vi "state_detect.vi"() -> ()   [LabVIEW 2012]
uses:
  <vilib>/DAQmx/create/channels.llb/DAQmx Create Channel (CO-Pulse Generation-Frequency).vi
  <vilib>/DAQmx/configure/timing.llb/DAQmx Timing (Implicit).vi
  <vilib>/Utility/file.llb/Write To Spreadsheet File (DBL).vi
  <vilib>/Analysis/NI_AALBase.lvlib
panel:
  in  "Save data to":path
  out "Fluorescence Before":T1(graph)
  out "Run Number":i32
  out "Total fluorescence with pumping":u32
  out "Total fluorescence without pumping":u32
  out "Optical pumping":bool
  out "Not_opt_pump_dark_runs":i32
  out "opt_pump_dark_runs":i32
  in  "Fluoresence Threshold":u32
  out "No_opt_pump_dark_run_ratio":dbl
  out "Opt_pump_Dark_run_ratio":dbl
  out "Fluorescence After":T2(graph)
  in  "Runs":i32
  in  "stop":bool
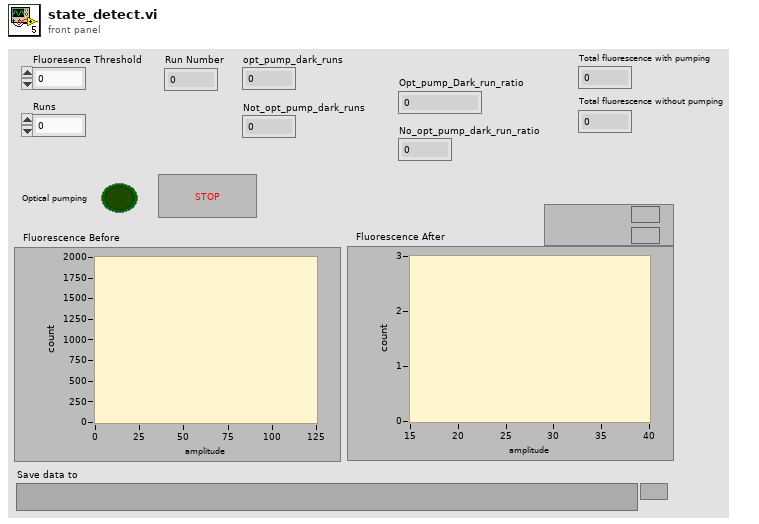
[diagram p1: front panel]
types:
  T1 = cluster{"X Values":dbl[], "Histogram: h(x)":i32[]}
  T2 = cluster{"X Values":dbl[], "Histogram: h(x)":i32[]}[]
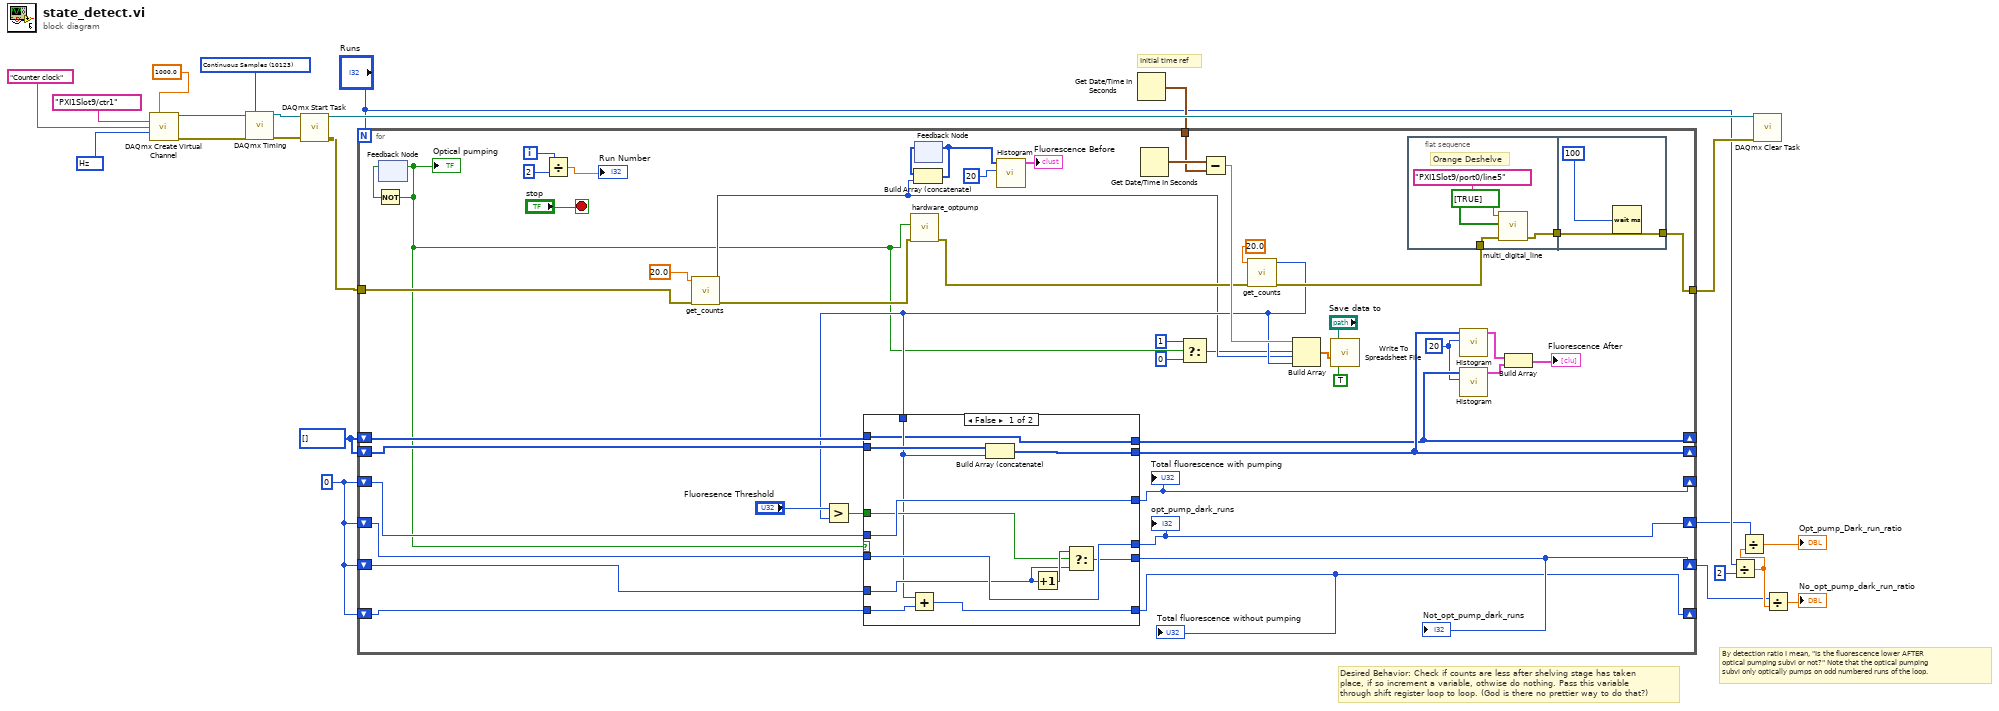
[diagram p0: block diagram]
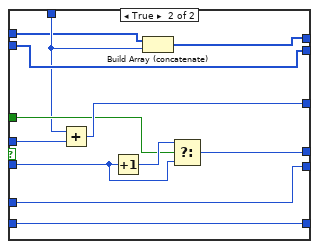
[diagram p2: hidden frame]
diagram:
  w2 = i32[] [] ("initialized array")
  w1 = 0
  w17 = 10123 items=["Finite Samples"=10178, "Continuous Samples"=10123, "Hardware Timed Single Point"=12522] ("sample mode")
  w22 = 10373 items=["Hz"=10373] ("units")
  # "Desired Behavior: Check if counts are less after shelving stage has taken\nplace, if so increment a variable, othwise do nothing. Pass this variable\nthrough shift register loop to loop. (God is there no prettier way to do that?)"
  # "Initial time ref"
  # "By detection ratio I mean, \"Is the fluorescence lower AFTER\noptical pumping subvi or not?\" Note that the optical pumping\nsubvi only optically pumps on odd numbered runs of the loop."
  n1 = call-poly <vilib>:"DAQmx Create Virtual Channel.vi"("frequency"=1000.0 ("rate"), "counter"=tag "PXI1Slot9/ctr1", "name to assign"="Counter clock", "units"=w22) -> ("task out"=w21:refnum<k21>, "error out"=w20:errorcluster)  [unwired: 10 in]
  n2 = call-poly <vilib>:"DAQmx Timing.vi"("task/channels in"=w21, "sample mode"=w17, "error in"=w20) -> ("task out"=w19:refnum<k21>, "error out"=w18:errorcluster)  [unwired: 11 in]
  n3 = call <vilib>:"DAQmx Start Task.vi"("task/channels in"=w19, "error in"=w18) -> ("task out"=w12:refnum<k21>, "error out"=w13:errorcluster)  [unwired: 12 in]
  n4 = Get Date/Time In Seconds() -> (seconds since 1Jan1904=w11:timestamp)
  n5 = for {
    N: "Runs" -> [_]
    tunnel: w13 -> [w63]
    tunnel: w11 -> [w66]
    tunnel: [w59] -> w10
    shift-right: [w42] -> _
    shift-left: w2 -> [w43]
    shift-right: [w40] -> _
    shift-left: w2 -> [w41]
    shift-right: [w55] -> w5
    shift-left: w1 -> [w62]
    shift-right: [w54] -> w7
    shift-left: w1 -> [w61]
    shift-right: [w50] -> _
    shift-left: w1 -> [w52]
    shift-right: [w51] -> _
    shift-left: w1 -> [w53]
    i -> [w48]
    stop <- "stop" stop-if-true
    w39 = 20 ("intervals")
    n6 = feedback #1() -> (w46:bool)  [unwired: 1 in]
    n7 = Not(x=w46) -> (.not. x?=w30:bool)
    "Optical pumping" <- w30
    n8 = feedback-in #1(w30) -> ()
    n9 = Divide(x=w48, y=2) -> (x/y=→"Run Number":dbl)
    n10 = call "get_counts.vi"("error in"=w63, "Detection length (ms)"=20.0) -> ("error out"=w57:errorcluster, "Counts"=w31:u32)  [unwired: 8 in]
    n11 = call "hardware_optpump.vi"("error in"=w57, "Pump?"=w30) -> ("error out"=w56:errorcluster)  [unwired: 9 in]
    n12 = feedback #2() -> (w35:u32[])  [unwired: 1 in]
    n13 = Build Array (concatenate)(w35, w31) -> (w23:u32[])
    n14 = feedback-in #2(w23) -> ()
    n15 = call <vilib>:"Histogram.vi"("intervals"=20, "X"=w23) -> ("Histogram Graph"=→"Fluorescence Before":T1)  [unwired: 6 in, 3 out]
    n16 = Get Date/Time In Seconds() -> (seconds since 1Jan1904=w67:timestamp)
    n17 = Select(t=1, s=w30, f=0) -> (s? t:f=w27:i32)
    n18 = Subtract(x=w67, y=w66) -> (x-y=w65:dbl)
    n19 = call "get_counts.vi"("error in"=w56, "Detection length (ms)"=20.0) -> ("error out"=w60:errorcluster, "Counts"=w32:u32)  [unwired: 8 in]
    n20 = Greater?(x="Fluoresence Threshold", y=w32) -> (0:w44:bool)
    n21 = case shown="False" w30 {
      tunnel: w62 -> [w82 w99]
      tunnel: w61 -> [w87 w94]
      tunnel: [w81 w99] -> w55
      tunnel: [w87 w93] -> w54
      tunnel: w32 -> [w78 w89]
      tunnel: w52 -> [w86 w98]
      tunnel: [w85 w98] -> w50
      tunnel: w53 -> [w84 w97]
      tunnel: [w84 w96] -> w51
      tunnel: w44 -> [w80 w92]
      tunnel: w43 -> [w79 w90]
      tunnel: [w77 w90] -> w42
      tunnel: [w76 w91] -> w40
      tunnel: w41 -> [w76 w88]
      frame False {
        n22 = Add(x=w78, y=w86) -> (x+y=w85:u32)
        n23 = Build Array (concatenate)(w79, w78) -> (w77:u32[])
        n24 = Increment(x=w82) -> (x+1=w83:i32)
        n25 = Select(t=w83, s=w80, f=w82) -> (s? t:f=w81:i32)
      }
      frame True {
        n26 = Add(x=w89, y=w97) -> (x+y=w96:u32)
        n27 = Increment(x=w94) -> (x+1=w95:i32)
        n28 = Build Array (concatenate)(w88, w89) -> (w91:u32[])
        n29 = Select(t=w95, s=w92, f=w94) -> (s? t:f=w93:i32)
      }
    }
    "opt_pump_dark_runs" <- w54
    "Not_opt_pump_dark_runs" <- w55
    "Total fluorescence with pumping" <- w51
    "Total fluorescence without pumping" <- w50
    n30 = Build Array(w65, w27, w31, w32) -> (w26:dbl[])
    n31 = call-poly <vilib>:"Write To Spreadsheet File.vi"("append to file? (new file:F)"=TRUE, "1D data"=w26, "file path (dialog if empty)"="Save data to") -> ()  [unwired: 5 in, 1 out]
    n32 = flat-sequence {
      tunnel: w60 -> [w73]
      tunnel: [w70] -> w58
      tunnel: [w75] -> w59
      tunnel: w58 -> [w75]
      frame #0 {
        # "Orange Deshelve"
        n33 = call "multi_digital_line.vi"("error in"=w73, "data"=bool[] [TRUE], "lines"=tag "PXI1Slot9/port0/line5" ("lines 2")) -> ("error out"=w70:errorcluster)  [unwired: 8 in]
      }
      frame #1 {
        n34 = Wait (ms)(milliseconds to wait=u32 100 ("455 Pumping Time 2")) -> ()  [unwired: 1 out]
      }
    }
    n35 = call <vilib>:"Histogram.vi"("intervals"=w39, "X"=w42) -> ("Histogram Graph"=w38:T1)  [unwired: 6 in, 3 out]
    n36 = call <vilib>:"Histogram.vi"("intervals"=w39, "X"=w40) -> ("Histogram Graph"=w37:T1)  [unwired: 6 in, 3 out]
    n37 = Build Array(w38, w37) -> (→"Fluorescence After":T2)
  }
  n38 = Divide(x="Runs", y=2) -> (x/y=w6:dbl)
  n39 = Divide(x=w7, y=w6) -> (x/y=→"Opt_pump_Dark_run_ratio":dbl)
  n40 = call <vilib>:"DAQmx Clear Task.vi"("task in"=w12, "error in"=w10) -> ()  [unwired: 13 in, 1 out]
  n41 = Divide(x=w5, y=w6) -> (x/y=→"No_opt_pump_dark_run_ratio":dbl)
